vi "nD Nonlinear System Prep (VI).vi"(6 "data":variant, 7 "F(X)":T2, 8 "h":dbl, 9 "accuracy":dbl, 10 "Diagonal h":T1, 11 "Start":dbl[](array[numeric])) -> (0 "error":i32, 1 "error":bool, 2 "F(X)":dbl[](array[numeric]), 3 "Start New":dbl[](array[numeric]))   [LabVIEW 2014, in "NI_Gmath.lvlib"]
uses:
  NI_Gmath.lvlib
  functionRefnum nD.ctl
  RealMatrix.ctl
  A x Vector.vi
  Unit Vector (DBL).vi
  Real Inverse Matrix.vi
  NI_AALBase.lvlib
  NI_Matrix.lvlib
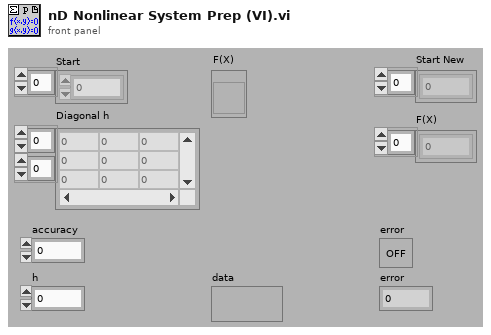
[diagram p1: front panel]
types:
  T1 = typedef "NI_Matrix.lvlib/RealMatrix.ctl" = dbl[][]
  T2 = typedef "NI_Gmath.lvlib/functionRefnum nD.ctl" = refnum<vi>
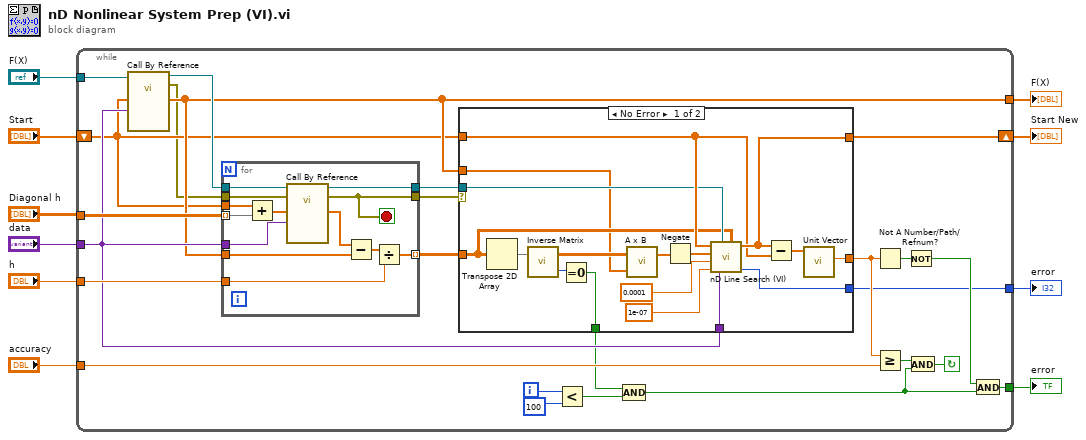
[diagram p0: block diagram]
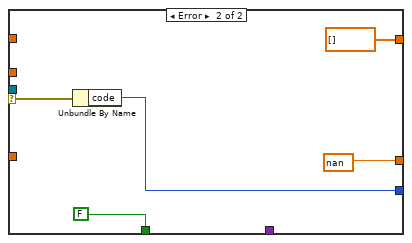
[diagram p2: hidden frame]
diagram:
  n1 = while {
    tunnel: [w27] -> w10
    tunnel: [w15] -> w5
    tunnel: "accuracy" -> [w33]
    tunnel: "h" -> [w34]
    shift-left: "Start" -> [w12]
    shift-right: [w22] -> w6
    tunnel: "F(X)" -> [w21]
    tunnel: "data" -> [w20]
    tunnel: "Diagonal h" -> [w35]
    tunnel: [w13] -> w8
    i -> [w29]
    stop <- w31 continue-if-true
    n2 = call-by-ref "?"(reference=w21, "variant"=w20, "X"=w12) -> (reference out=w18:T2, error out=w11:errorcluster, 2:"F(X)"=w15:dbl[])  [unwired: 4 in]
    n3 = for {
      tunnel: w35 -> [w70] mode=indexing
      tunnel: w34 -> [w68]
      tunnel: [w65] -> w16 mode=indexing
      tunnel: w18 -> [w64]
      tunnel: w20 -> [w63]
      tunnel: w12 -> [w69]
      tunnel: w15 -> [w66]
      tunnel: [w60] -> w17
      tunnel: w11 -> [w59]
      tunnel: [w58] -> w14
      stop <- w58 stop-if-true
      n4 = Add(x=w69, y=w70) -> (x+y=w62:dbl[])
      n5 = call-by-ref "?"(reference=w64, error in=w59, "variant"=w63, "X"=w62) -> (reference out=w60:T2, error out=w58:errorcluster, 2:"F(X)"=w61:dbl[])  [unwired: 3 in]
      n6 = Subtract(x=w61, y=w66) -> (x-y=w67:dbl[])
      n7 = Divide(x=w67, y=w68) -> (x/y=w65:dbl[])
    }
    n8 = case shown="No Error" w14 {
      selector: w14 -> [_ w55]
      tunnel: [w45 nan] -> w25
      tunnel: [w44 dbl[] [] ("X (new)")] -> w22
      tunnel: w20 -> [w42 _]
      tunnel: w12 -> [w41 _]
      tunnel: [w40 FALSE] -> w19
      tunnel: w17 -> [w39 _]
      tunnel: w16 -> [w38 _]
      tunnel: w15 -> [w36 _]
      tunnel: [w37 w54] -> w13
      frame No Error {
        n9 = Transpose 2D Array(2D array=w38) -> (transposed array=w47:dbl[][])
        n10 = call-poly "Inverse Matrix.vi"("Input Matrix"=w47) -> ("error"=w46:i32, "Inverse Matrix"=w52:T1)  [unwired: 1 in]
        n11 = Equal To 0?(x=w46) -> (x = 0?=w40:bool)
        n12 = call-poly "A x B.vi"("Vector"=w36, "A"=w52) -> ("A x Vector"=w51:dbl[])  [unwired: 1 out]
        n13 = Negate(x=w51) -> (-x=w50:dbl[])
        n14 = call "nD Line Search (VI).vi"("J"=w38, "data"=w42, "F(X)"=w39, "TOLX"=1e-07, "alpha"=0.0001, "P"=w50, "X"=w41) -> ("error"=w37:i32, "X (new)"=w44:dbl[])  [unwired: 3 out]
        n15 = Subtract(x=w44, y=w41) -> (x-y=w43:dbl[])
        n16 = call-poly "Unit Vector.vi"("Input Vector"=w43) -> ("norm"=w45:dbl)  [unwired: 2 in, 8 out]
      }
      frame Error {
        n17 = Unbundle By Name(w55) -> ("code"=w54:i32)
      }
    }
    n18 = Less?(x=w29, y=100) -> (x < y?=w30:bool)
    n19 = Compound Arithmetic op=AND(w19, w30) -> (w28:bool)
    n20 = Not A Number/Path/Refnum?(number/path/refnum=w25) -> (NaN/Path/Refnum?=w24:bool)
    n21 = Greater Or Equal?(x=w25, y=w33) -> (x >= y?=w26:bool)
    n22 = Not(x=w24) -> (.not. x?=w23:bool)
    n23 = And(x=w26, y=w28) -> (x .and. y?=w31:bool)
    n24 = And(x=w23, y=w28) -> (x .and. y?=w27:bool)
  }
  "error" <- w10
  "error" <- w8
  "Start New" <- w6
  "F(X)" <- w5
